vi "findGetParamsHelper.vi"(0 "params in":refnum<class "JSON Value.lvclass">, 1 "outputDataDictionary":refnum<class "data dictionary.lvclass">, 11 "error in":errorcluster) -> (3 "tagindex":i32, 4 "params out":refnum<class "JSON Value.lvclass">, 6 "tagname":string, 8 "tagtype":T1, 13 "missingParam":string, 14 "invalidTagType":string, 15 "error out":errorcluster)   [LabVIEW 2018, in "JSON_RPC_Interface runtime.lvclass"]
uses:
  JSON_RPC_Interface runtime.lvclass
  <vilib>/NI/JSON Support for LabVIEW/JSON Value/JSON Value.lvclass
  <vilib>/NI/Tag Bus/tag/Data Type.ctl
  <vilib>/NI/Tag Bus/dictionary/data dictionary.lvclass
  <vilib>/NI/JSON Support for LabVIEW/JSON Value/Read Value/Read value (String).vi
  <vilib>/NI/Tag Bus/tag/tag descriptor.lvclass
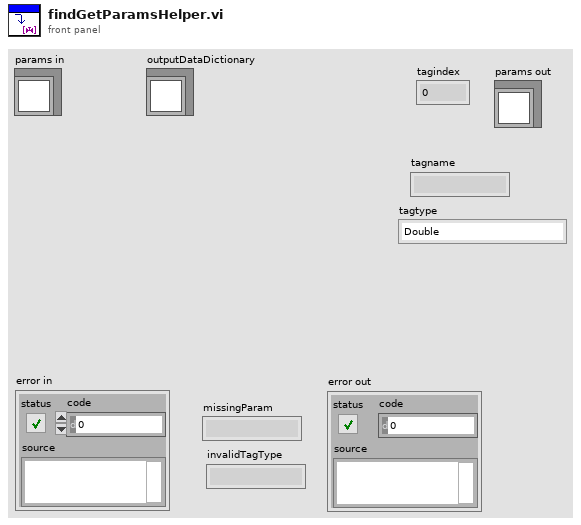
[diagram p1: front panel]
types:
  T1 = typedef "tag bus.lvlib/tag descriptor.lvclass/Data Type.ctl" = enum16{"Double", "Single", "I64", "I32", "I16", "I8", "U64", "U32", "U16", "U8", "Boolean", "String", "Array of Double", "Array of Single", "Array of I64", "Array of I32", "Array of I16", "Array of I8", "Array of U64", "Array of U32", "Array of U16", "Array of U8", "Array of Boolean", "Array of String"}
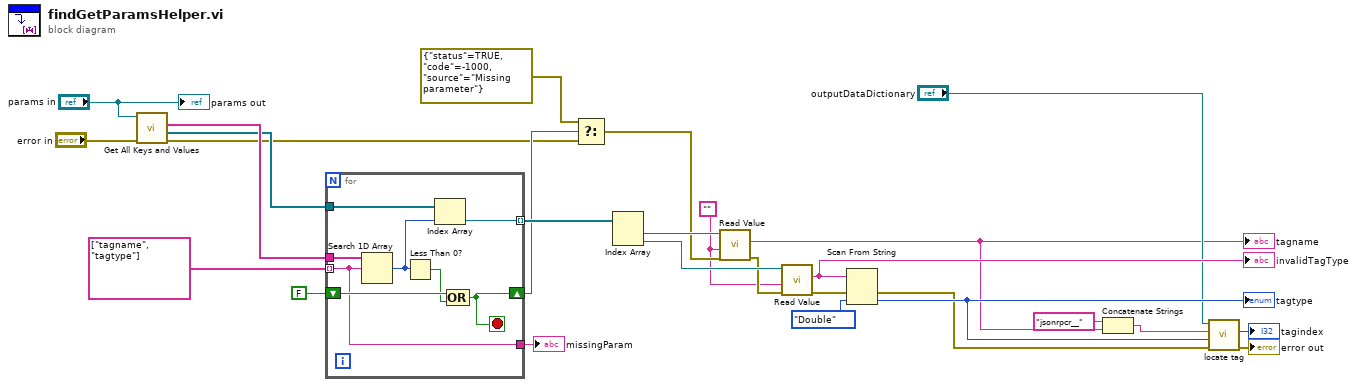
[diagram p0: block diagram]
diagram:
  w12 = ""
  n1 = call <vilib>:"Get All Keys and Values.vi"("error in"="error in", "JSON Value in"="params in") -> ("error out"=w16:errorcluster, "values"=w21:refnum<class "JSON Value.lvclass">[], "keys"=w26:string[])  [unwired: 7 in]
  n2 = for {
    tunnel: w26 -> [w35]
    tunnel: w21 -> [w30]
    tunnel: string[] ["tagname", "tagtype"] -> [w31] mode=indexing
    shift-right: [w32] -> w17
    shift-left: FALSE -> [w34]
    tunnel: [w31] -> w13
    tunnel: [w28] -> w18 mode=indexing
    stop <- w32 stop-if-true
    n3 = Search 1D Array(1D array=w35, element=w31) -> (index of element=w29:i32)  [unwired: 1 in]
    n4 = Less Than 0?(x=w29) -> (x < 0?=w33:bool)
    n5 = Index Array(array=w30, index=w29) -> (element=w28:refnum<class "JSON Value.lvclass">)
    n6 = Compound Arithmetic op=OR(w34, w33) -> (w32:bool)
  }
  "missingParam" <- w13
  n7 = Select(t=errorcluster {"status"=TRUE, "code"=-1000, "source"="Missing parameter"}, s=w17, f=w16) -> (s? t:f=w15:errorcluster)
  n8 = Index Array(array=w18) -> (element #1=w24:refnum<class "JSON Value.lvclass">, element #2=w23:refnum<class "JSON Value.lvclass">)  [unwired: 2 in]
  n9 = call-poly <vilib>:"Read Value.vi"("error in (no error)"=w15, "default value"=w12, "JSON String in"=w24) -> ("error out"=w22:errorcluster, "value"=w2:string)  [unwired: 6 in, 1 out]
  "tagname" <- w2
  n10 = call-poly <vilib>:"Read Value.vi"("error in (no error)"=w22, "default value"=w12, "JSON String in"=w23) -> ("error out"=w10:errorcluster, "value"=w9:string)  [unwired: 6 in, 1 out]
  "invalidTagType" <- w9
  n11 = Scan From String(input string=w9, error in=w10, default 1=Data_Type."Double" ("Data Type")) -> (error out=w4:errorcluster, output 1=w8:T1)  [unwired: 2 in, 2 out]
  "tagtype" <- w8
  n12 = Concatenate Strings("jsonrpcr__" ("string"), w2) -> (w3:string)
  n13 = call <vilib>:"locate tag.vi"("error in"=w4, "data type"=w8, "name"=w3, "data dictionary in"="outputDataDictionary") -> ("error out"=→"error out":errorcluster, "index"=→"tagindex":i32)  [unwired: 5 in, 1 out]
  "params out" <- "params in"
